vi "Ping - Get stats.vi"(11 "Ping Output":string) -> (1 "# of packets received":i32, 2 "# of packets sent":i32, 3 "IP Address":string)   [LabVIEW 2013]
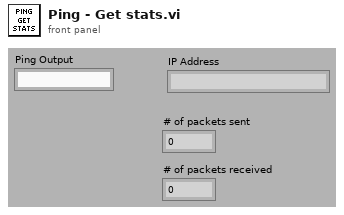
[diagram p1: front panel]
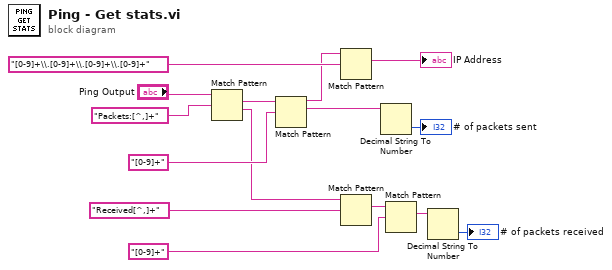
[diagram p0: block diagram]
diagram:
  n1 = Match Pattern(string="Ping Output", regular expression="Packets:[^,]+" ("regular expression 2")) -> (match substring=w11:string, after substring=w1:string)  [unwired: 3 out]
  n2 = Match Pattern(string=w11, regular expression="[0-9]+") -> (before substring=w13:string, match substring=w2:string)  [unwired: 3 out]
  n3 = Match Pattern(string=w13, regular expression="[0-9]+\\.[0-9]+\\.[0-9]+\\.[0-9]+") -> (match substring=→"IP Address":string)  [unwired: 4 out]
  n4 = Match Pattern(string=w1, regular expression="Received[^,]+") -> (match substring=w5:string)  [unwired: 4 out]
  n5 = Decimal String To Number(string=w2) -> (number=→"# of packets sent":i32)  [unwired: 3 out]
  n6 = Match Pattern(string=w5, regular expression="[0-9]+") -> (match substring=w3:string)  [unwired: 4 out]
  n7 = Decimal String To Number(string=w3) -> (number=→"# of packets received":i32)  [unwired: 3 out]
